vi "Append Properties To Edit Context Menu.vi"(9 "State":T1, 11 "Menu in":refnum<k9>) -> ()   [LabVIEW 2020, in "Noise (G3).xctl"]
uses:
  Noise (G3).xctl
  State.ctl
  Noise (G3) - Persistent.ctl
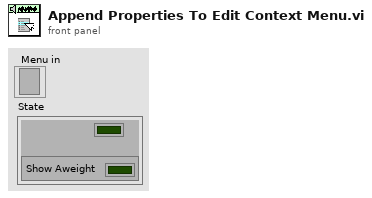
[diagram p1: front panel]
types:
  T1 = typedef "Noise (G3).xctl/State.ctl" = cluster{"enable menu":bool, "persistent":T2}
  T2 = typedef "Noise (G3).xctl/Noise (G3) - Persistent.ctl" = cluster{"Show Aweight":bool}
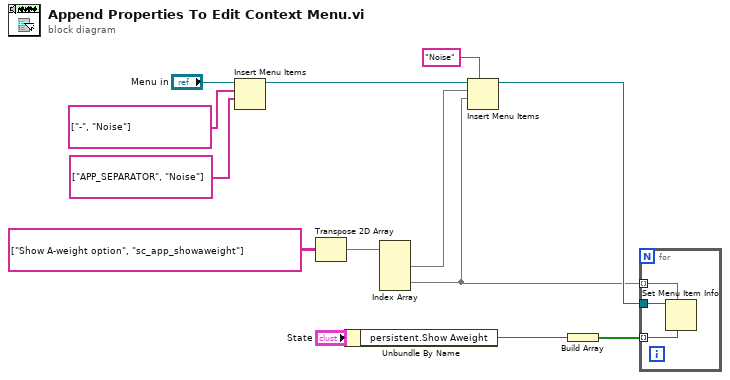
[diagram p0: block diagram]
diagram:
  n1 = Insert Menu Items(7:string[] ["APP_SEPARATOR", "Noise"] ("item names"), 8:string[] ["-", "Noise"] ("item names"), 9:"Menu in") -> (3:w12:refnum<k9>)  [unwired: 3 in, 2 out]
  n2 = Transpose 2D Array(2D array=string[][] [["Show A-weight option", "sc_app_showaweight"]] ("item names")) -> (transposed array=w7:string[][])
  n3 = Unbundle By Name("State") -> ("persistent.Show Aweight"=w4:bool)
  n4 = Index Array(array=w7) -> (element #1=w6:string[], element #2=w1:string[])  [unwired: 4 in]
  n5 = Insert Menu Items(5:"Noise", 7:w1, 8:w6, 9:w12) -> (3:w2:refnum<k9>)  [unwired: 2 in, 2 out]
  n6 = Build Array(w4) -> (w3:bool[])
  n7 = for {
    tunnel: w2 -> [w16]
    tunnel: w3 -> [w15] mode=indexing
    tunnel: w1 -> [w14] mode=indexing
    n8 = Set Menu Item Info(6:w15, 7:w14, 11:w16) -> ()  [unwired: 4 in, 2 out]
  }
